vi "XIPIN_AHB-Lite_to_AXI_Bridge_3_0.vi"   [LabVIEW 2017]
doc: "Connects AXI slave with AHB-Lite masters\n------------------------------------\n<b>Need License</b> : No\n<b>Interface</b> : AXI4"
uses:
  <vilib>/rvi/XilinxIP/XIPIN_XNode/niFpgaXIPIN.xnode
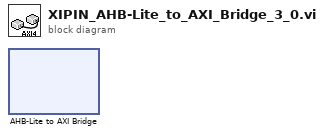
[diagram p0: block diagram]
diagram:
  n1 = xnode ("AHB-Lite to AXI Bridge")() -> ()
